vi "MQTT Connection Properties.vi"(9 "Connect Flags":T2={"user name"=TRUE, "password"=FALSE, "will retain"=FALSE, "will flag"=FALSE, "clean session"=FALSE, "reserved"=FALSE, "will QoS"=enum."At most once"}, 10 "Client ID":string="LabVIEW_MQTT_Client", 11 "User Info":T1={"User Name"="06A543AQfC3DorkicfpL", "Password"=""}) -> (2 "output cluster":T6)   [LabVIEW 2014]
uses:
  LVMQTT-master/Controls/QoS.ctl
  LVMQTT-master/Controls/DUP_Flag.ctl
  LVMQTT-master/Controls/Retain_Flag.ctl
  LVMQTT-master/Controls/Connect_Flags.ctl
  LVMQTT-master/Controls/User_Info.ctl
  LVMQTT-master/MQTT_Functions.lvlib
panel:
  in  "MQTT Broker":cluster{"address (IP)":string, "port":u16}={"address (IP)"="things.ktk.gubkin.ru", "port"=1883}
  in  "Connect Meta":T7={"QoS"=enum."At most once", "DUP"=FALSE, "Retain"=FALSE, "Keep Alive (sec)"=60}
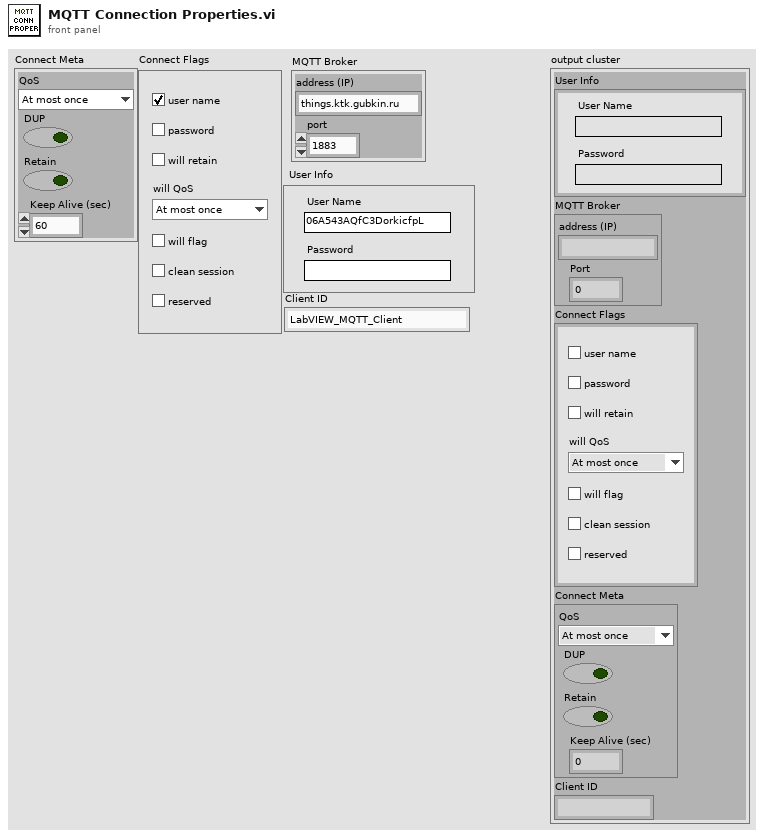
[diagram p1: front panel]
types:
  T1 = typedef "MQTT_Functions.lvlib/User_Info.ctl" = cluster{"User Name":string, "Password":string}
  T2 = typedef "MQTT_Functions.lvlib/Connect_Flags.ctl" = cluster{"user name":bool, "password":bool, "will retain":bool, "will flag":bool, "clean session":bool, "reserved":bool, "will QoS":T3}
  T3 = typedef "MQTT_Functions.lvlib/QoS.ctl" = enum8{"At most once", "At least once", "Exactly once", "Reserved"}
  T4 = typedef "MQTT_Functions.lvlib/DUP_Flag.ctl" = bool
  T5 = typedef "MQTT_Functions.lvlib/Retain_Flag.ctl" = bool
  T6 = cluster{"User Info":T1, "MQTT Broker":cluster{"address (IP)":string, "Port":i32}, "Connect Flags":T2, "Connect Meta":cluster{"QoS":T3, "DUP":T4, "Retain":T5, "Keep Alive (sec)":u16}, "Client ID":string}
  T7 = cluster{"QoS":T3, "DUP":T4, "Retain":T5, "Keep Alive (sec)":u16}
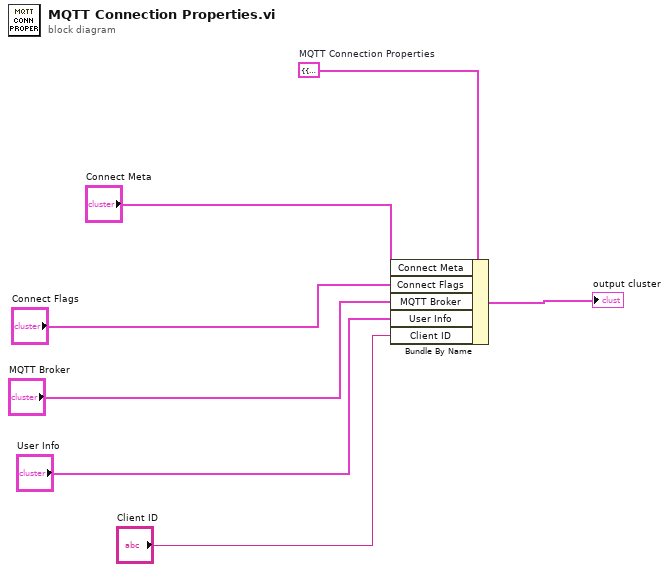
[diagram p0: block diagram]
diagram:
  w2 = T6 {"User Info"={"User Name"="", "Password"=""}, "MQTT Broker"={"address (IP)"="", "Port"=0}, "Connect Flags"={"user name"=FALSE, "password"=FALSE, "will retain"=FALSE, "will flag"=FALSE, "clean session"=FALSE, "reserved"=FALSE, "will QoS"=enum."At most once"}, "Connect Meta"={"QoS"=enum."At most once", "DUP"=FALSE, "Retain"=FALSE, "Keep Alive (sec)"=60}, "Client ID"=""}  # MQTT Connection Properties
  n1 = Bundle By Name(cluster=w2, "Connect Meta"="Connect Meta", "Connect Flags"="Connect Flags", "MQTT Broker"="MQTT Broker", "User Info"="User Info", "Client ID"="Client ID") -> (→"output cluster":T6)
